vi "acquireValue.vi"(8 "error in (no error)":errorcluster, 10 "nextSample?":bool, 11 "setDigitalFilter in":refnum<class "setDigitalFilter.lvclass">) -> (0 "error out":errorcluster, 1 "function return":i32, 2 "variantData":variant, 3 "setDigitalFilter out":refnum<class "setDigitalFilter.lvclass">)   [LabVIEW 2016, in "SALLV_MtAtElectrometer_Messaging.lvlib" / "setDigitalFilter.lvclass"]
uses:
  setDigitalFilter.lvclass
  ts_sallv_MtAtElectrometer/SALLV_MtAtElectrometer.lvlib
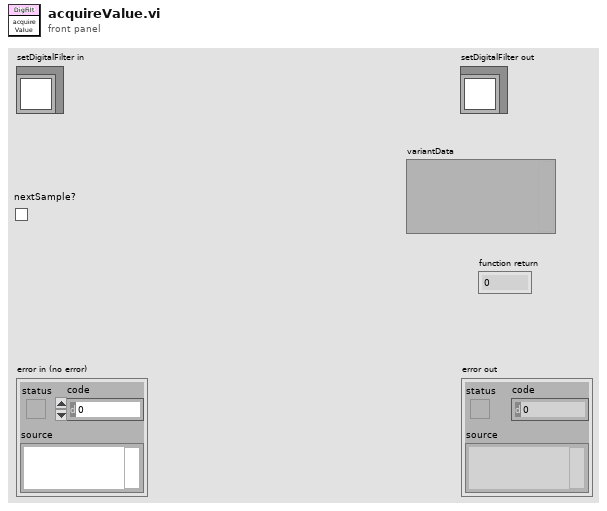
[diagram p1: front panel]
types:
  T1 = typedef "SALLV_MtAtElectrometer.lvlib/command_setDigitalFilter.ctl" = cluster{"activateFilter":bool, "averageFilter":u16, "medianFilter":bool}
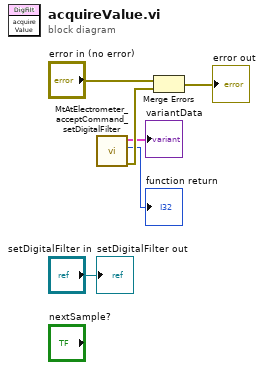
[diagram p0: block diagram]
diagram:
  n1 = call "MtAtElectrometer_acceptCommand_setDigitalFilter.vi"() -> ("error out"=w3:errorcluster, "function return"=→"function return":i32, "command_setDigitalFilter_Ctl out"=→"variantData":T1)  [unwired: 9 in]
  n2 = Merge Errors("error in (no error)", w3) -> (→"error out":errorcluster)
  "setDigitalFilter out" <- "setDigitalFilter in"
